vi "猜拳.vi"() -> ()   [LabVIEW 2016]
uses:
  Controls/robotdata.ctl
  D:/Program Files (x86)/National Instruments/LabVIEW 2016/vi.lib/MakerHub/Leap/Private/Libs/LeapCSharp.NET3.5.dll
  Program Files (x86)/National Instruments/LabVIEW 2016/vi.lib/MakerHub/Leap/Private/Libs/LeapCSharp.NET3.5.dll
  <vilib>/Utility/miscctls.llb/LVRGBAColorTypeDef.ctl
  <vilib>/LabVIEW Interface for Arduino/LabVIEW Interface for Arduino.lvlib
panel:
  out "Count":i32
  out "IsEmpty":bool
  in  "错误输入（无错误）":errorcluster
  out "错误输出":errorcluster
  in  "背景色":u32(colorbox)=15204350
  in  "转    台：":sgl(slide) scale=0.0..90.0 scale format="%#_g°"
  in  "手    臂：":sgl(slide) scale=0.0..90.0 scale format="%#_g°"
  in  "上下移动：":dbl(slide)=6.46551724137931 scale=0.0..100.0
  in  "拇指":sgl(slide) caption="拇    指：" scale=0.0..60.0 scale format="%#_g°"
  in  "食    指：":sgl(slide) caption="食指" scale=0.0..90.0 scale format="%#_g°"
  in  "中    指：":sgl(slide) caption="中指" scale=0.0..90.0 scale format="%#_g°"
  in  "无名指：":sgl(slide) caption="无名指" scale=0.0..90.0 scale format="%#_g°"
  in  "小手指：":sgl(slide) caption="小手指" scale=0.0..90.0 scale format="%#_g°"
  in  "手    腕：":sgl(slide) scale=0.0..90.0 scale format="%#_g°"
  in  "hand":T1={"手腕"=52.38806, "小手指"=0.0, "无名指"=0.0, "中指"=0.0, "食指"=0.0, "上下移动"=-1.8918918918918917, "背景色"=15204350, "拇指"=0.0, "转台"=52.38806, "手臂"=52.38806} {"手臂" scale=0.0..90.0; "转台" scale=0.0..360.0; "拇指" scale=0.0..90.0; "上下移动" scale=0.0..100.0; "食指" scale=0.0..90.0; "中指" scale=0.0..90.0; "无名指" scale=0.0..90.0; "小手指" scale=0.0..90.0; "手腕" scale=0.0..360.0}
  out "机械手":refnum<vi>(3d-picture)
  in  "退出":bool=TRUE
  # "创世捷能 CSJN"
  # "趣味机械手"
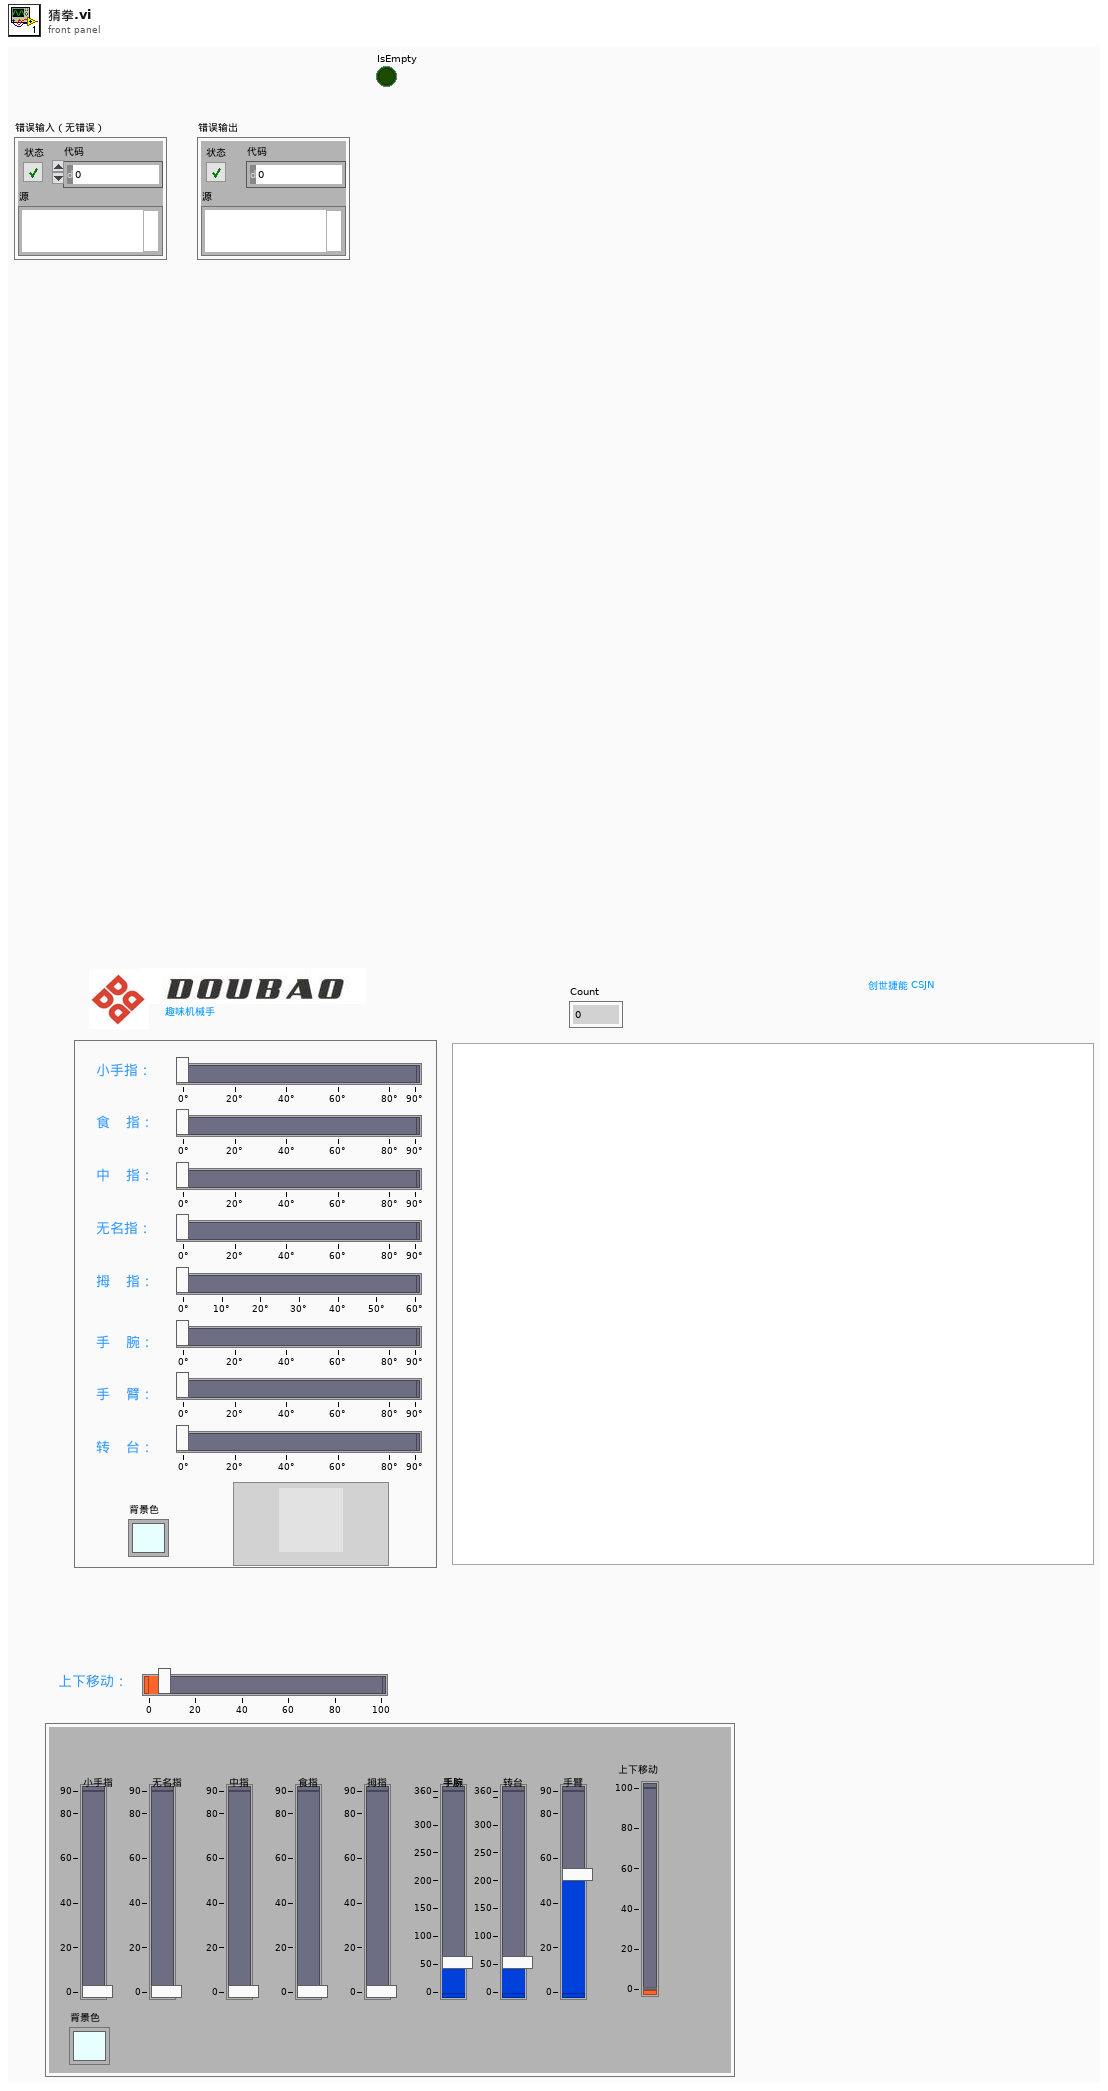
[diagram p1: front panel]
types:
  T1 = typedef "robotdata.ctl" = cluster{"手腕":sgl, "小手指":sgl, "无名指":sgl, "中指":sgl, "食指":sgl, "上下移动":dbl, "背景色":u32, "拇指":sgl, "转台":sgl, "手臂":sgl}
  T2 = enum16{"石头", "剪刀", "布", "你赢了", "你输了", "再来一局", "NAN"}
  T3 = typedef "LabVIEW Interface for Arduino.lvlib/Arduino Resource.ctl" = cluster{"VISA resource":refnum<visa-resource-name>, "Board Type":T4, "Connection Type":enum8{"USB / Serial"}, "Bytes Per Packet (15)":u8}
  T4 = typedef "LabVIEW Interface for Arduino.lvlib/Board Type.ctl" = enum16{"Uno", "Dimuelanove w/Atmega 328", "Mega 2560"}
  T5 = typedef "handdata.ctl" = cluster{"机械手":refnum<vi>, "转台":refnum<vi>, "手臂":refnum<vi>, "手腕":refnum<vi>, "拇指指尖":refnum<vi>, "拇指指中 ":refnum<vi>, "食指指中":refnum<vi>, "食指指尖":refnum<vi>, "中指指中":refnum<vi>, "中指指尖":refnum<vi>, "无名指指中":refnum<vi>, "无名指指尖":refnum<vi>, "小手指指中":refnum<vi>, "小手指指尖":refnum<vi>}
  T6 = typedef "LVRGBAColorTypeDef.ctl" = cluster{"Red":sgl, "Green":sgl, "Blue":sgl, "Alpha":sgl}
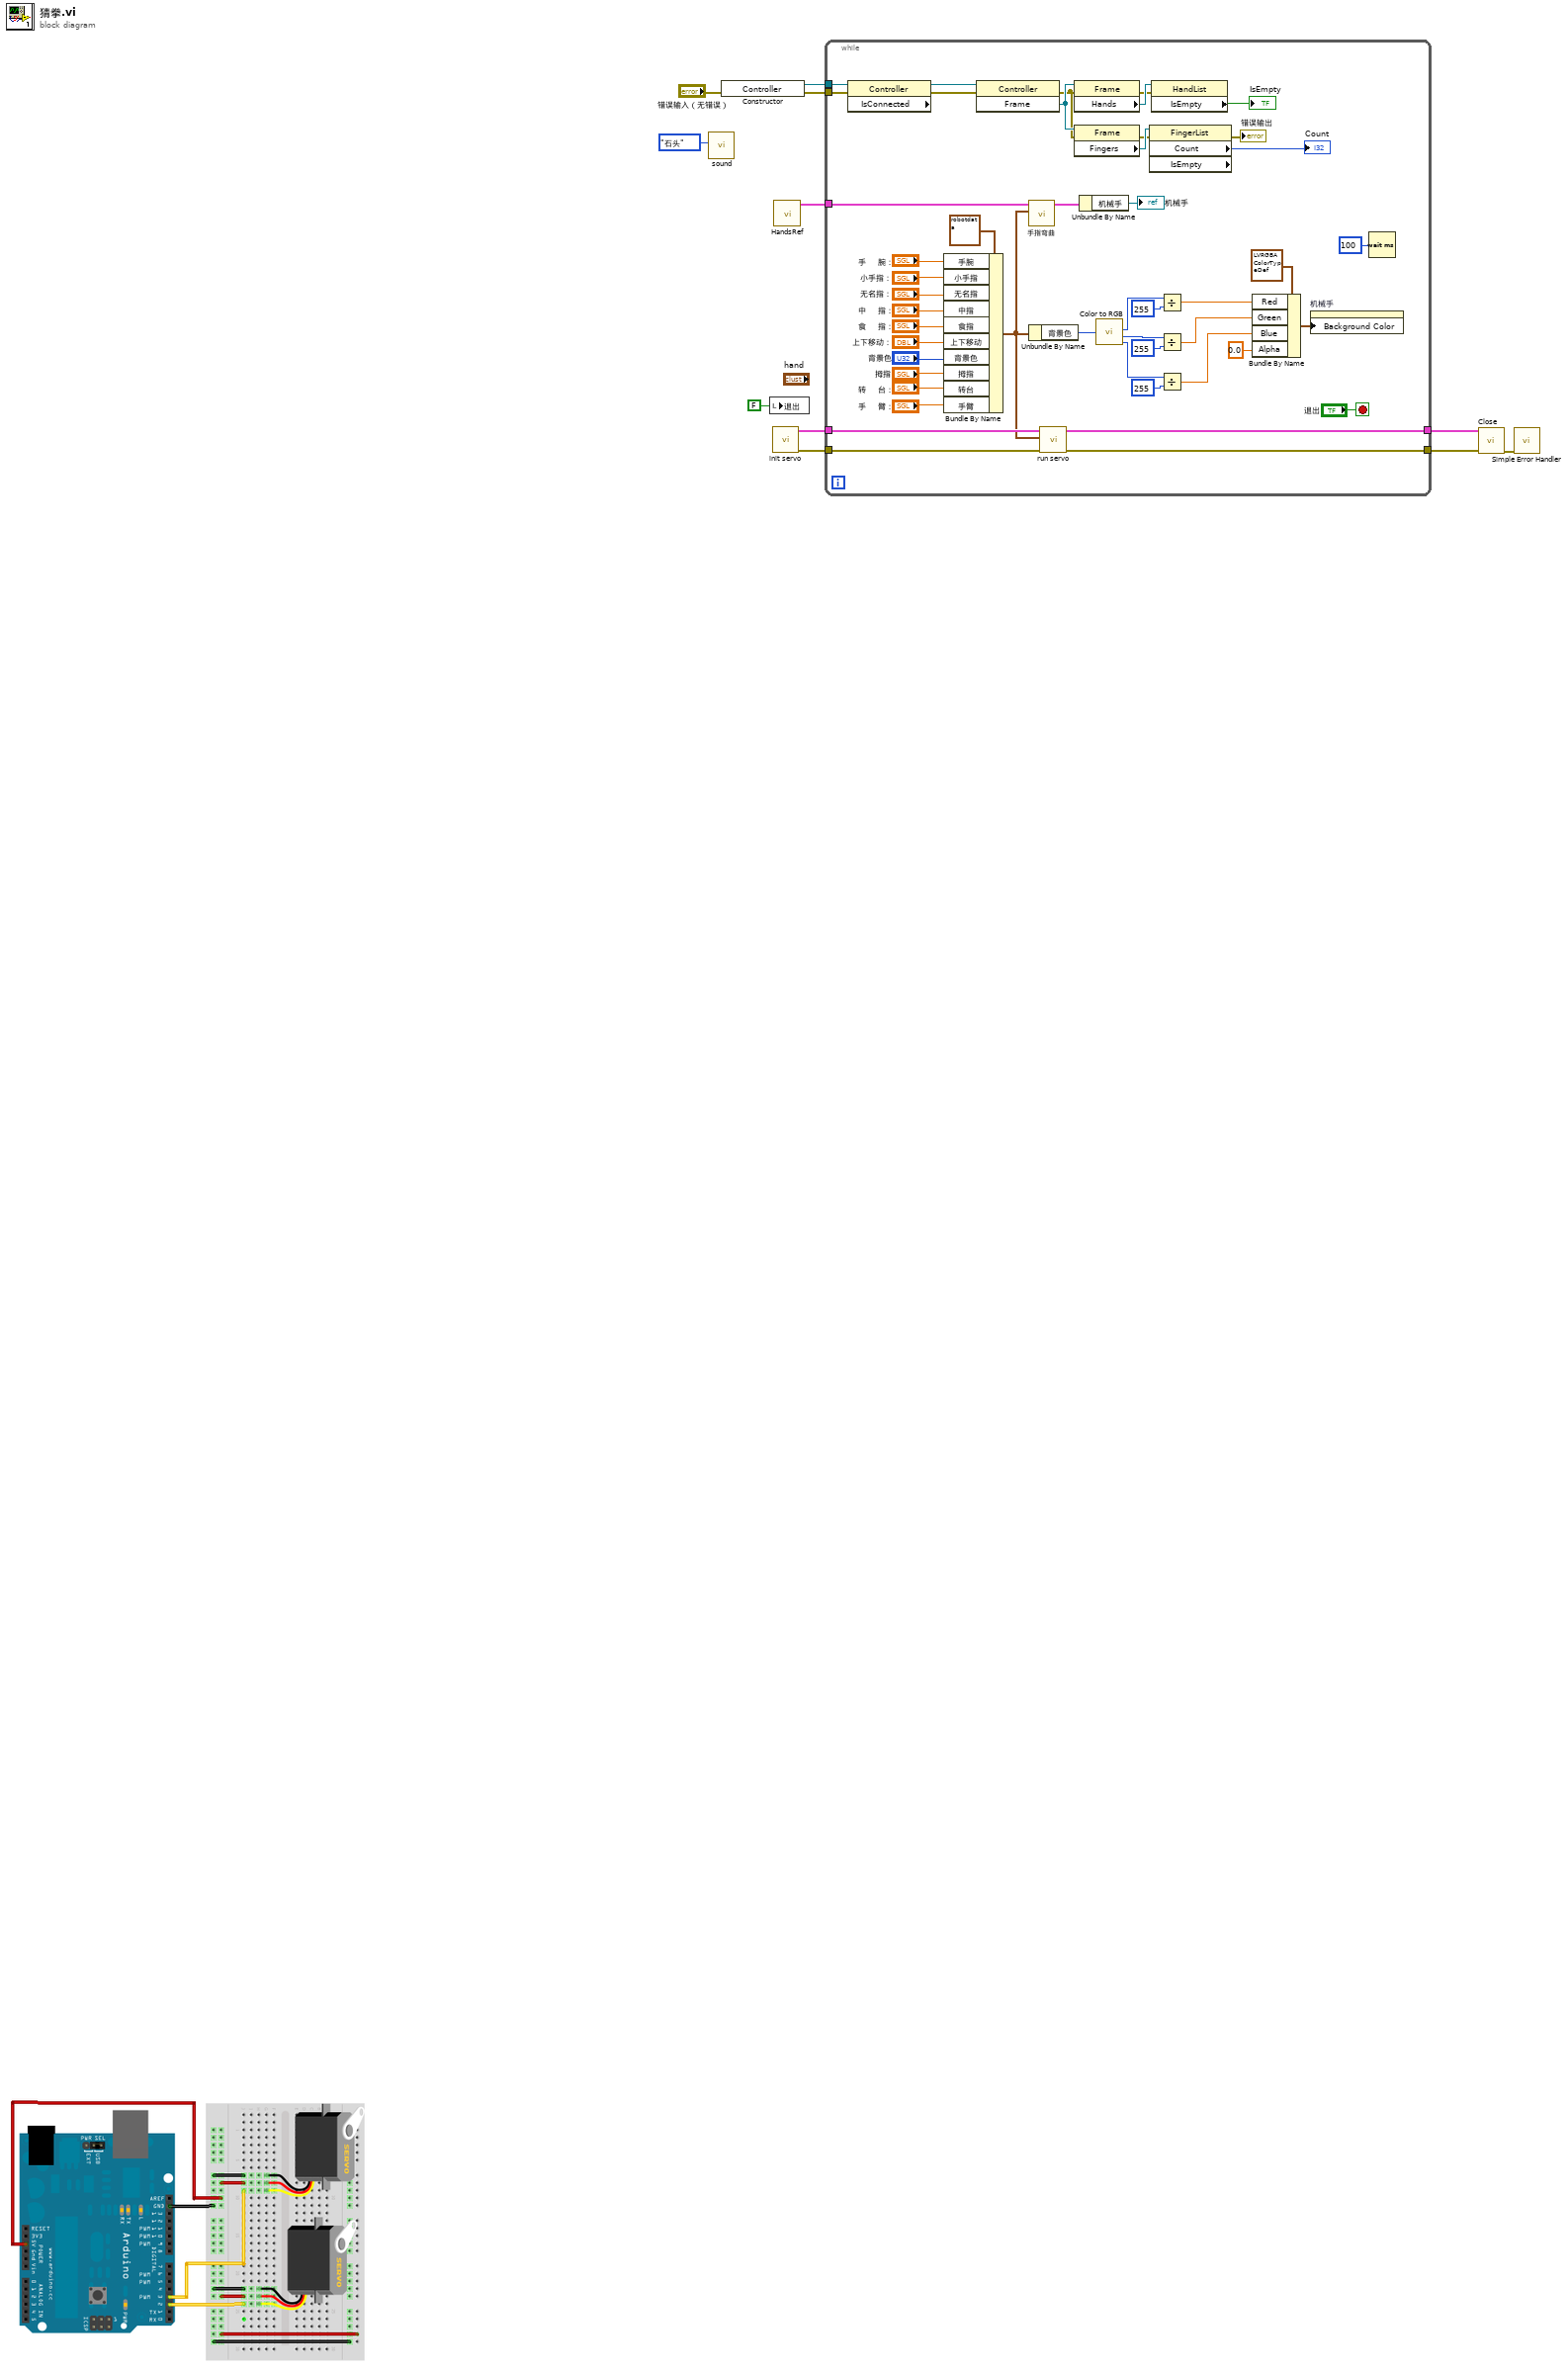
[diagram p0: block diagram]
diagram:
  n1 = call "sound.vi"("sound"=T2."石头") -> ()  [unwired: 10 in, 1 out]
  n2 = constructor class="Controller"(error in="错误输入（无错误）") -> (reference out=w3:refnum<k24>, error out=w2:errorcluster)  [unwired: 2 in, 1 out]
  n3 = local write "退出"(FALSE ("退出")) -> ()
  n4 = call "init servo.vi"() -> ("错误输出"=w7:errorcluster, "Arduino Resource"=w9:T3)  [unwired: 10 in]
  n5 = call "HandsRef.vi"() -> ("簇"=w10:T5)  [unwired: 9 in, 2 out]
  n6 = while {
    tunnel: w10 -> [w44]
    tunnel: w9 -> [w29]
    tunnel: [w28] -> w8
    tunnel: w7 -> [w27]
    tunnel: [w26] -> w6
    tunnel: w3 -> [w15]
    tunnel: w2 -> [w13]
    stop <- "退出" stop-if-true
    n7 = property class="Controller" props=["IsConnected"](reference=w15, error in=w13) -> (reference out=w24:refnum<k24>, error out=w14:errorcluster)  [unwired: 1 out]
    n8 = Bundle By Name(cluster=T1 {"手腕"=52.38806, "小手指"=0.0, "无名指"=0.0, "中指"=0.0, "食指"=0.0, "上下移动"=-1.8918918918918917, "背景色"=15204350, "拇指"=0.0, "转台"=52.38806, "手臂"=52.38806} ("hand"), "手腕"="手    腕：", "小手指"="小手指：", "无名指"="无名指：", "中指"="中    指：", "食指"="食    指：", "上下移动"="上下移动：", "背景色"="背景色", "拇指"="拇指", "转台"="转    台：", "手臂"="手    臂：") -> (w25:T1)
    n9 = invoke class="Controller" method="Frame"(reference=w24, error in=w14) -> (error out=w19:errorcluster, "Frame"=w20:refnum<k24>)  [unwired: 1 in, 1 out]
    n10 = call "手指弯曲.vi"("Hands Data In"=w25, "Hands Ref In"=w44) -> ("Hands Ref Out"=w43:T5)  [unwired: 7 in, 2 out]
    n11 = Unbundle By Name(w25) -> ("背景色"=w46:u32)
    n12 = call "run servo.vi"("错误输入（无错误）"=w27, "hand"=w25, "Arduino Resource输入"=w29) -> ("错误输出"=w26:errorcluster, "Arduino Resource输出"=w28:T3)  [unwired: 7 in]
    n13 = property class="Frame"(reference=w20, error in=w19) -> (error out=w17:errorcluster, "Hands"=w18:refnum<k24>)  [unwired: 1 out]
    n14 = property class="Frame"(reference=w20, error in=w19) -> (error out=w16:errorcluster, "Fingers"=w23:refnum<k24>)  [unwired: 1 out]
    n15 = Unbundle By Name(w43) -> ("机械手"=→"机械手":refnum<vi>)
    n16 = call <vilib>:"Color to RGB.vi"("Color"=w46) -> ("R"=w50:u8, "G"=w51:u8, "B"=w47:u8)  [unwired: 1 out]
    n17 = property class="FingerList" props=["Count", "IsEmpty"](reference=w23, error in=w16) -> (error out=→"错误输出":errorcluster, "Count"=→"Count":i32)  [unwired: 2 out]
    n18 = property class="HandList"(reference=w18, error in=w17) -> ("IsEmpty"=→"IsEmpty":bool)  [unwired: 2 out]
    n19 = Divide(x=w50, y=u32 255) -> (x/y=w55:dbl)
    n20 = Divide(x=w51, y=u32 255) -> (x/y=w52:dbl)
    n21 = Divide(x=w47, y=u32 255) -> (x/y=w48:dbl)
    n22 = Bundle By Name(cluster=T6 {"Red"=0.7, "Green"=0.7, "Blue"=0.7, "Alpha"=0.0} ("背景色"), "Red"=w55, "Green"=w52, "Blue"=w48, "Alpha"=sgl 0.0) -> (w58:T6)
    n23 = property on="机械手" class="SceneGraphDisp (严格)"("Background Color"=w58) -> ()  [unwired: 2 in, 2 out]
    n24 = Wait (ms)(milliseconds to wait=u32 100 ("等待时间（毫秒）")) -> ()  [unwired: 1 out]
  }
  n25 = call <vilib>:"Close.vi"("Arduino Resource"=w8, "error in"=w6) -> ("error out"=w5:errorcluster)  [unwired: 13 in]
  n26 = call <vilib>:"Simple Error Handler.vi"("error in (no error)"=w5) -> ()  [unwired: 4 in, 5 out]
